vi "Start Scan.vi"(8 "error in (no error)":errorcluster, 11 "PF_API in":refnum<class "PF_API.lvclass">) -> (0 "error out":errorcluster, 3 "PF_API out":refnum<class "PF_API.lvclass">)   [LabVIEW 2019, in "PF_API.lvclass"]
doc: "Sends a command to start the Scan Stream."
uses:
  PF_API.lvclass
  PF_API.lvclass/PF_API.ctl
  <vilib>/httpClient/POSTBuffer.vi
  <vilib>/httpClient/LabVIEWHTTPClient.lvlib
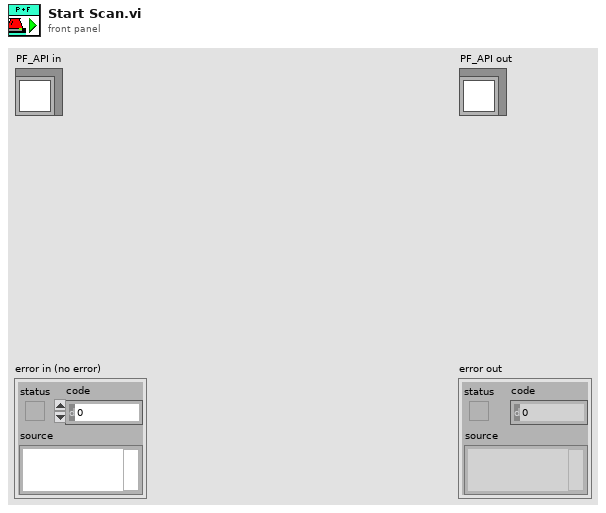
[diagram p1: front panel]
types:
  T1 = typedef "LabVIEWHTTPClient.lvlib/ClientHandle.ctl" = refnum<k1>
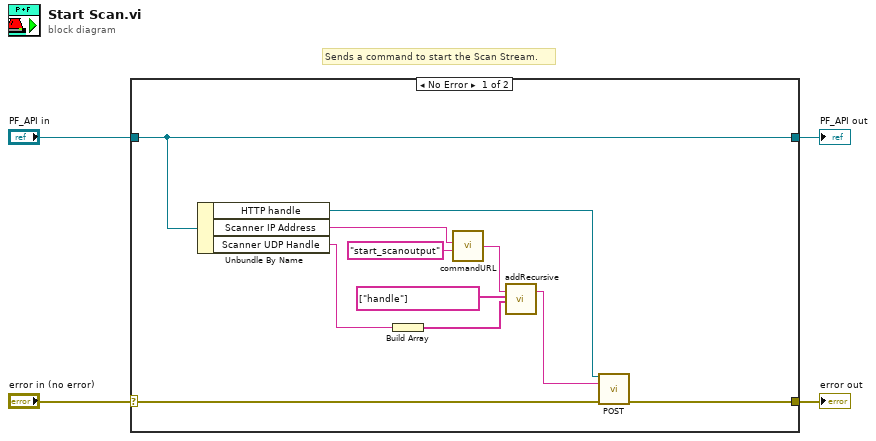
[diagram p0: block diagram]
diagram:
  # "Sends a command to start the Scan Stream."
  n1 = case shown="No Error" "error in (no error)" {
    selector: "error in (no error)" -> [w15 w17]
    tunnel: [w13 w17] -> w3
    tunnel: [w14 w16] -> w1
    tunnel: "PF_API in" -> [w14 w16]
    frame No Error {
      n2 = Unbundle By Name(w14) -> ("HTTP handle"=w12:T1, "Scanner IP Address"=w11:string, "Scanner UDP Handle"=w7:string)
      n3 = Build Array(w7) -> (w6:string[])
      n4 = call "commandURL.vi"("Command String"="start_scanoutput", "Scanner IP Address"=w11) -> ("Command URL"=w9:string)  [unwired: 4 in]
      n5 = call "addRecursive.vi"("Command URL in"=w9, "Parameter Key"=string[] ["handle"], "Parameter Value"=w6) -> ("Command URL out"=w5:string)  [unwired: 13 in, 3 out]
      n6 = call-poly <vilib>:"POST.vi"("client handle"=w12, "url"=w5, "error in (no error)"=w15) -> ("error out"=w13:errorcluster)  [unwired: 9 in, 3 out]
    }
    frame Error {
    }
  }
  "error out" <- w3
  "PF_API out" <- w1
